vi "F Dwf Analog In Frequency Info.vi"(8 "error in (no error)":errorcluster, 9 "phzMax":dbl, 10 "phzMin":dbl, 11 "hdwf":i32) -> (0 "error out":errorcluster, 1 "phzMax out":dbl, 2 "phzMin out":dbl, 3 "function return":i32)   [LabVIEW 2019, in "Olasdwf.lvlib"]
doc: "DWFAPI int FDwfAnalogInFrequencyInfo(HDWF hdwf, double *phzMin, double *phzMax);"
uses:
  Olasdwf.lvlib
  Windows/System32/dwf.dll
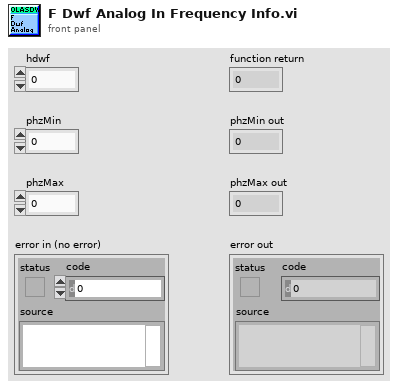
[diagram p1: front panel]
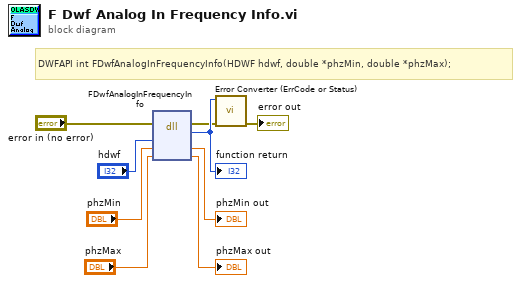
[diagram p0: block diagram]
diagram:
  # "DWFAPI int FDwfAnalogInFrequencyInfo(HDWF hdwf, double *phzMin, double *phzMax);"
  n1 = dll-call lib="C:/Windows/System32/dwf.*" fn="FDwfAnalogInFrequencyInfo"(error in="error in (no error)", "hdwf"="hdwf", "phzMin"="phzMin", "phzMax"="phzMax") -> (error out=w2:errorcluster, w9:i32, "phzMin"=→"phzMin out":dbl, "phzMax"=→"phzMax out":dbl)  [unwired: 3 in, 1 out]
  "function return" <- w9
  n2 = call "Error Converter (ErrCode or Status).vi"("error in (no error)"=w2, "error code"=w9) -> ("error out"=→"error out":errorcluster)  [unwired: 9 in]
